vi "CloseAll.vi"(8 "error in (no error)":errorcluster) -> (0 "error out":errorcluster)   [LabVIEW 2017, in "UI.lvlib"]
doc: "Write data to main coms q for module (generic)"
uses:
  UI.lvlib
  ctl/MainData.ctl
  ctl/MainStates.ctl
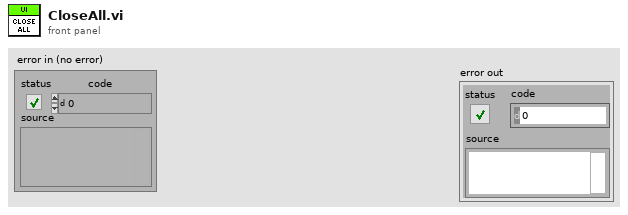
[diagram p1: front panel]
types:
  T1 = typedef "UI.lvlib/MainStates.ctl" = enum16{"Timeout", "Error", "Exit", "Init", "UpdatePrice", "CloseAll"}
  T2 = typedef "UI.lvlib/MainData.ctl" = cluster{"State":T1, "Variant":variant}
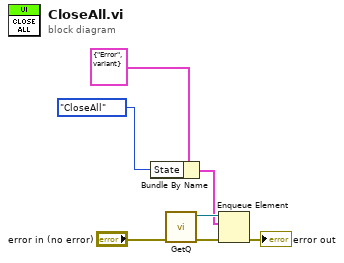
[diagram p0: block diagram]
diagram:
  n1 = Bundle By Name(cluster=T2 {"State"=enum."Error", "Variant"=variant} ("Data"), "State"=MainStates."CloseAll") -> (w3:T2)
  n2 = call "GetQ.vi"("error in (no error)"="error in (no error)") -> ("error out"=w6:errorcluster, "Q out"=w7:refnum<queue>)  [unwired: 9 in]
  n3 = Enqueue Element(queue=w7, element=w3, error in (no error)=w6) -> (error out=→"error out":errorcluster)  [unwired: 1 in, 2 out]
